vi "PGResetCameraWait.vi"(6 "Extra Waits":i32, 7 "Cycle time\n(ms)":i32=3 min=0 step=1, 8 "error in":errorcluster, 9 "BIN":u16(ring) items=["1x1", "2x2", "4x4"], 10 "MODE":u16(ring) items=["Normal", "DIF"], 11 "VISA resource name":refnum<visa-resource-name>) -> (0 "error out":errorcluster, 3 "VISA resource name out":refnum<visa-resource-name>)   [LabVIEW 2018]
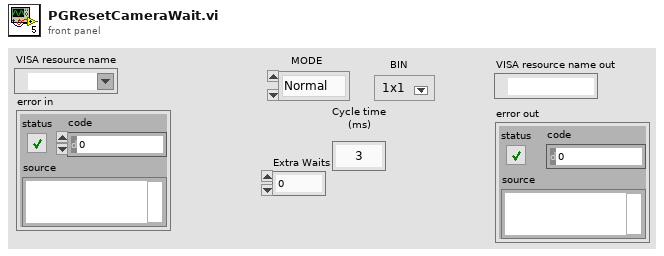
[diagram p1: front panel]
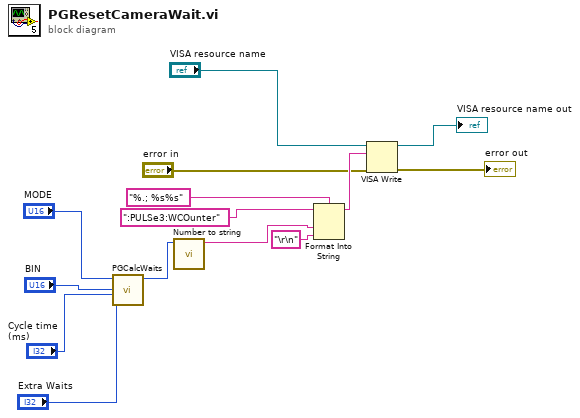
[diagram p0: block diagram]
diagram:
  n1 = call "PGCalcWaits.vi"("Extra Waits"="Extra Waits", "Cycle time\n(ms)"="Cycle time\n(ms)", "BIN"="BIN", "MODE"="MODE") -> ("Wait"=w5:i32)  [unwired: 7 in]
  n2 = call "Number to string.vi"("Numeric"=w5) -> ("Shortest String"=w12:string)  [unwired: 10 in]
  n3 = Format Into String(format string="%.; %s%s", initial string=":PULSe3:WCOunter" ("format string"), w12, "\r\n" ("format string")) -> (resulting string=w10:string)  [unwired: 1 in, 1 out]
  n4 = VISA Write(VISA resource name="VISA resource name", write buffer=w10, error in (no error)="error in") -> (VISA resource name out=→"VISA resource name out":refnum<visa-resource-name>, error out=→"error out":errorcluster)  [unwired: 1 out]
